vi "실습 2-11 2D Vector 모션.vi"() -> ()   [LabVIEW 2014]
uses:
  <vilib>/Motion/FlexMotion/CustomControls/CustomControls.llb/AxisOrVectorSpace To Configure.flx
  <vilib>/Motion/FlexMotion/FunctionsVIs/StartStopMotion.llb/Start Motion (8 axes).flx
  <vilib>/Motion/FlexMotion/FunctionsVIs/Trajectory.llb/Check Move Complete Status (8 axes).flx
  <vilib>/Motion/FlexMotion/FunctionsVIs/StartStopMotion.llb/Stop Motion (8 axes).flx
panel:
  in  "Z Position (0)":i32
  in  "Y Position (0)":i32
  in  "X Position (0)":i32
  in  "정지":bool
  out "Position":i32
  in  "Velocity (10000)":i32=3600
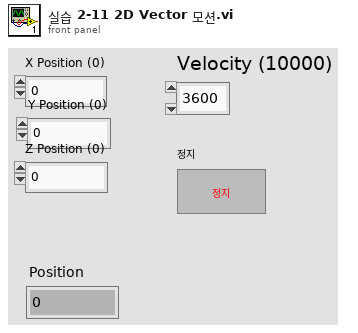
[diagram p1: front panel]
types:
  T1 = enum16{"None", "Axis 1", "Axis 2", "Axis 3", "Axis 4", "Axis 5", "Axis 6", "Axis 7", "Axis 8"}
  T2 = enum16{"Absolute Position", "Relative Position", "Velocity", "Relative to Cap Pos", "Modulus Position", "Absolute Contouring", "Relative Contouring"}
  T3 = typedef "AxisOrVectorSpace To Configure.flx" = u16
  T4 = typedef "Resource Out (Enum).flx" = u16
  T5 = typedef "Bd Id Out" = u8
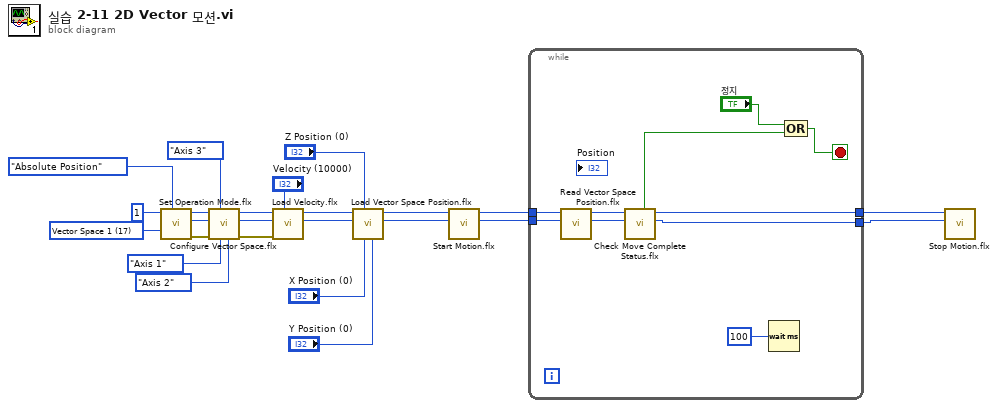
[diagram p0: block diagram]
diagram:
  w23 = T3 17 items=["Axis 1"=1, "Axis 2"=2, "Axis 3"=3, "Axis 4"=4, "Axis 5"=5, "Axis 6"=6, "Axis 7"=7, "Axis 8"=8, "Vector Space 1"=17, "Vector Space 2"=18, "Vector Space 3"=19, "Vector Space 4"=20] ("Axis or Vector Space")
  n1 = call <vilib>:"Set Operation Mode.flx"("Position Mode (Absolute)"=T2."Absolute Position", "Axis or Vector Space"=w23, "Board ID"=u8 1) -> ("error out"=w16:errorcluster, "Resource Output"=w17:T4, "Bd ID Out"=w18:T5)  [unwired: 3 in]
  n2 = call <vilib>:"Configure Vector Space.flx"("Y Axis (2)"=T1."Axis 2", "X Axis (1)"=T1."Axis 1", "Z Axis (3)"=T1."Axis 3", "error in (no error)"=w16, "Vector Space"=w17, "Board ID"=w18) -> ("error out"=w10:errorcluster, "Resource Output"=w11:T4, "Bd ID Out"=w12:T5)  [unwired: 3 in]
  n3 = call <vilib>:"Load Velocity.flx"("Velocity (10000)"="Velocity (10000)", "error in (no error)"=w10, "Axis or Vector Space"=w11, "Board ID"=w12) -> ("Resource Output"=w8:T4, "Bd ID Out"=w9:T5)  [unwired: 3 in, 1 out]
  n4 = call <vilib>:"Load Vector Space Position.flx"("Y Position (0)"="Y Position (0)", "X Position (0)"="X Position (0)", "Z Position (0)"="Z Position (0)", "Vector Space"=w8, "Board ID"=w9) -> ("Resource Output"=w3:T4, "Bd ID Out"=w4:T5)  [unwired: 4 in, 1 out]
  n5 = call-poly <vilib>:"Start Motion.flx"("Axis or Vector Space"=w3, "Board ID"=w4) -> ("Resource Output"=w19:T4, "Bd ID Out"=w20:T5)  [unwired: 4 in, 1 out]
  n6 = while {
    tunnel: w20 -> [w31]
    tunnel: w19 -> [w30]
    tunnel: [w26] -> w2
    tunnel: [w25] -> w1
    stop <- w33 stop-if-true
    n7 = call <vilib>:"Read Vector Space Position.flx"("Vector Space"=w30, "Board ID"=w31) -> ("Resource Output"=w28:T4, "Bd ID Out"=w29:T5)  [unwired: 4 in, 4 out]
    n8 = call-poly <vilib>:"Check Move Complete Status.flx"("Axis or Vector Space"=w28, "Board ID"=w29) -> ("Resource Output"=w25:T4, "Bd ID Out"=w26:T5, "Move Complete"=w27:bool)  [unwired: 4 in, 1 out]
    n9 = Wait (ms)(milliseconds to wait=u32 100 ("대기 시간(ms)")) -> ()  [unwired: 1 out]
    n10 = Compound Arithmetic op=OR("정지", w27) -> (w33:bool)
  }
  n11 = call-poly <vilib>:"Stop Motion.flx"("Axis or Vector Space"=w1, "Board ID"=w2) -> ()  [unwired: 5 in, 3 out]
